vi "Read SubComponent Data - Scaled.vi"(8 "error in (no error)":errorcluster, 11 "Bus Monitor in":refnum<class "Bus Monitor.lvclass">) -> (0 "error out":errorcluster, 1 "Scaled Data":dbl[](array[numeric]), 2 "Parameter":string[](array[string]), 3 "Bus Monitor out":refnum<class "Bus Monitor.lvclass">)   [LabVIEW 2020, in "BCI-1553 API.lvlib" / "Bus Monitor.lvclass"]
doc: "Reads the scaled values transacted for the parameters defined in each filter."
uses:
  Bus Monitor.lvclass
  Bus Monitor.lvclass/Bus Monitor.ctl
  Dependencies/Registry/Registry.lvclass/Registry.ctl
  Filters/Filter/Filter.lvclass
  Dependencies/Registry/Registry.lvclass
  BCI-1553 API.lvlib
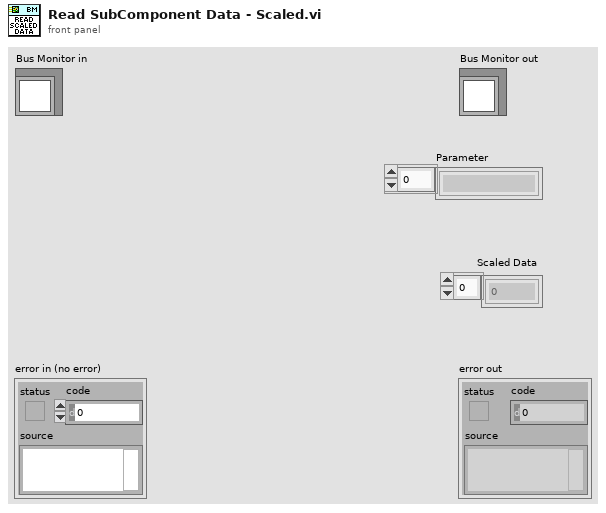
[diagram p1: front panel]
types:
  T1 = typedef "BCI-1553 API.lvlib/Parameter Table Data.ctl" = cluster{"Parameter Name":string, "Base Word":u16, "Address":u16, "Value":u64, "Mask":u16[], "Scaling Info":T2}
  T2 = typedef "BCI-1553 API.lvlib/Scaling Information.ctl" = cluster{"Bit Offset":i32, "Bit Count":i32, "LSB Resolution":dbl, "2's Complement":bool, "Big Endian":bool, "Sign Bit":bool}
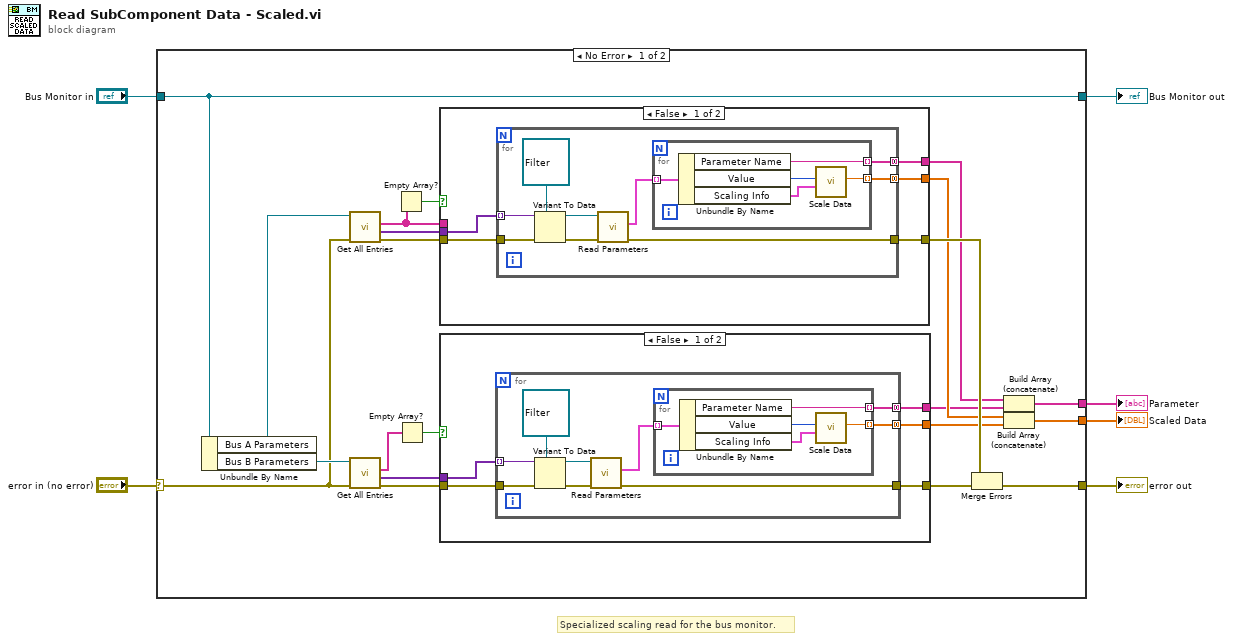
[diagram p0: block diagram]
diagram:
  # "Specialized scaling read for the bus monitor."
  n1 = case shown="No Error" "error in (no error)" {
    selector: "error in (no error)" -> [w12 w68]
    tunnel: "Bus Monitor in" -> [w11 w69]
    tunnel: [w19 w68] -> w4
    tunnel: [w14 _] -> w2
    tunnel: [w13 _] -> w1
    tunnel: [w11 w69] -> w3
    frame No Error {
      n2 = Unbundle By Name(w11) -> ("Bus A Parameters"=w27:refnum<class "Registry.lvclass">, "Bus B Parameters"=w26:refnum<class "Registry.lvclass">)
      n3 = call "Get All Entries.vi"("error in (no error)"=w12, "Registry in"=w27) -> ("error out"=w22:errorcluster, "Values"=w24:variant[], "Keys"=w10:string[])  [unwired: 7 in]
      n4 = call "Get All Entries.vi"("error in (no error)"=w12, "Registry in"=w26) -> ("error out"=w23:errorcluster, "Values"=w25:variant[], "Keys"=w8:string[])  [unwired: 7 in]
      n5 = Empty Array?(array=w10) -> (empty?=w9:bool)
      n6 = Empty Array?(array=w8) -> (empty?=w7:bool)
      n7 = case shown="False" w9 {
        tunnel: w24 -> [w52 _]
        tunnel: w22 -> [w51 w67]
        tunnel: [w50 w67] -> w20
        tunnel: [w49 _] -> w17
        tunnel: [w48 _] -> w15
        tunnel: w10 -> [_ _]
        frame False {
          n8 = for {
            tunnel: w52 -> [w60] mode=indexing
            tunnel: w51 -> [w61]
            tunnel: [w56] -> w50
            tunnel: [w54] -> w48 mode=concatenating
            tunnel: [w53] -> w49 mode=concatenating
            n9 = Variant To Data(error in=w61, type=refnum<class "Filter.lvclass"> refnum ("SLSC 1553 API.lvlib:Filter.lvclass"), Variant=w60) -> (data=w58:refnum<class "Filter.lvclass">, error out=w57:errorcluster)
            n10 = call-dynamic "Read Parameters.vi"("error in (no error)"=w57, "Filter in"=w58) -> ("error out"=w56:errorcluster, "Parameters"=w55:T1[])  [unwired: 7 in, 1 out]
            n11 = for {
              tunnel: [w66] -> w54 mode=indexing
              tunnel: [w64] -> w53 mode=indexing
              tunnel: w55 -> [w63] mode=indexing
              n12 = Unbundle By Name(w63) -> ("Parameter Name"=w66:string, "Value"=w65:u64, "Scaling Info"=w62:T2)
              n13 = call "Scale Data.vi"("Scaling Info"=w62, "Raw Value"=w65) -> ("Scaled Value"=w64:dbl)  [unwired: 8 in, 1 out]
            }
          }
        }
        frame True {
        }
      }
      n14 = case shown="False" w7 {
        tunnel: w25 -> [w32 _]
        tunnel: w23 -> [w31 w47]
        tunnel: [w30 w47] -> w21
        tunnel: [w29 _] -> w18
        tunnel: [w28 _] -> w16
        frame False {
          n15 = for {
            tunnel: w32 -> [w41] mode=indexing
            tunnel: w31 -> [w40]
            tunnel: [w36] -> w30
            tunnel: [w34] -> w28 mode=concatenating
            tunnel: [w33] -> w29 mode=concatenating
            n16 = Variant To Data(error in=w40, type=refnum<class "Filter.lvclass"> refnum ("SLSC 1553 API.lvlib:Filter.lvclass"), Variant=w41) -> (data=w38:refnum<class "Filter.lvclass">, error out=w37:errorcluster)
            n17 = call-dynamic "Read Parameters.vi"("error in (no error)"=w37, "Filter in"=w38) -> ("error out"=w36:errorcluster, "Parameters"=w35:T1[])  [unwired: 7 in, 1 out]
            n18 = for {
              tunnel: w35 -> [w46] mode=indexing
              tunnel: [w45] -> w34 mode=indexing
              tunnel: [w43] -> w33 mode=indexing
              n19 = Unbundle By Name(w46) -> ("Parameter Name"=w45:string, "Value"=w44:u64, "Scaling Info"=w42:T2)
              n20 = call "Scale Data.vi"("Scaling Info"=w42, "Raw Value"=w44) -> ("Scaled Value"=w43:dbl)  [unwired: 8 in, 1 out]
            }
          }
        }
        frame True {
        }
      }
      n21 = Merge Errors(w20, w21) -> (w19:errorcluster)
      n22 = Build Array (concatenate)(w15, w16) -> (w14:string[])
      n23 = Build Array (concatenate)(w17, w18) -> (w13:dbl[])
    }
    frame Error {
    }
  }
  "error out" <- w4
  "Bus Monitor out" <- w3
  "Scaled Data" <- w1
  "Parameter" <- w2
